vi "Log to Excel.vi"(8 "error in":errorcluster, 11 "tdms file in":refnum<k34>) -> (0 "error out":errorcluster, 2 "appended array":dbl[][][](array[numeric]), 3 "tdms file out":refnum<k34>)   [LabVIEW 2014, in "Logger.lvlib"]
uses:
  Logger.lvlib
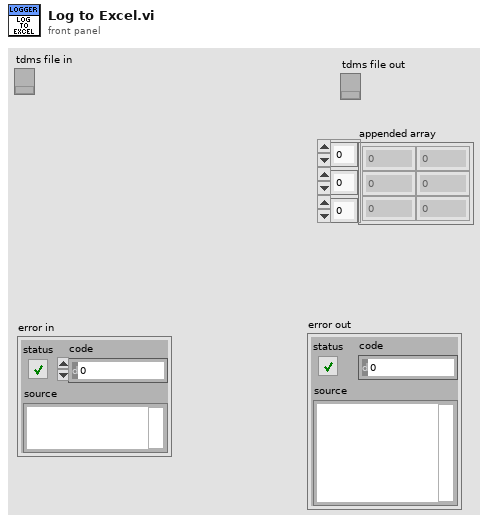
[diagram p1: front panel]
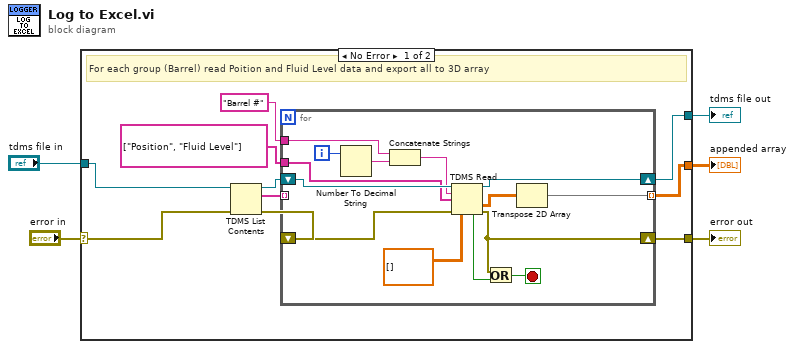
[diagram p0: block diagram]
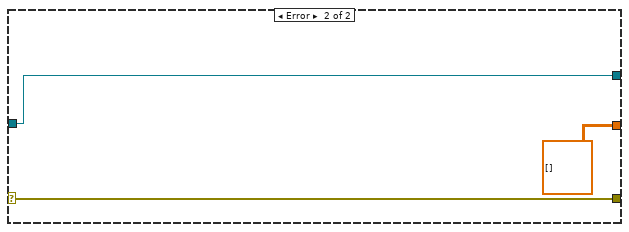
[diagram p2: hidden frame]
diagram:
  n1 = case shown="No Error" "error in" {
    selector: "error in" -> [w9 w32]
    tunnel: [w14 dbl[][][] []] -> w5
    tunnel: [w13 w32] -> w4
    tunnel: [w11 w31] -> w3
    tunnel: "tdms file in" -> [w6 w31]
    frame No Error {
      # "For each group (Barrel) read Poition and Fluid Level data and export all to 3D array"
      n2 = TDMS List Contents(4:w9, 7:w6) -> (0:w8:errorcluster, 2:w10:string[], 3:w7:refnum<k34>)  [unwired: 1 in, 1 out]
      n3 = for {
        tunnel: string[] ["Position", "Fluid Level"] -> [w21]
        tunnel: "Barrel #" -> [w26]
        tunnel: [w19] -> w14 mode=indexing
        shift-right: [w18] -> w13
        shift-left: w8 -> [w28]
        tunnel: w10 -> [_] mode=indexing
        shift-right: [w23] -> w11
        shift-left: w7 -> [w29]
        i -> [w24]
        stop <- w16 stop-if-true
        n4 = Number To Decimal String(number=w24) -> (decimal integer string=w25:string)  [unwired: 1 in]
        n5 = Concatenate Strings(w26, w25) -> (w22:string)
        n6 = TDMS Read(0:w29, 5:w22, 7:w21, 11:w28, 12:dbl[][] [] ("appended array")) -> (4:w23:refnum<k34>, 10:w20:dbl[][], 14:w17:bool, 15:w18:errorcluster)  [unwired: 3 in, 2 out]
        n7 = Or(x=w18, y=w17) -> (x .or. y?=w16:bool)
        n8 = Transpose 2D Array(2D array=w20) -> (transposed array=w19:dbl[][])
      }
    }
    frame Error {
    }
  }
  "error out" <- w4
  "appended array" <- w5
  "tdms file out" <- w3
